vi "SA_OUT.vi"(8 "error in (no error)":errorcluster, 10 "拍攝A讀取條碼":string, 11 "DBLink":string) -> (0 "error out":errorcluster, 2 "Workspace: screw_B":cluster{"條碼A":string, "條碼B":string}[](array[cluster]), 3 "Workspace: screw_A":cluster{"條碼A":string, "條碼B":string}[](array[cluster]))   [LabVIEW 2019]
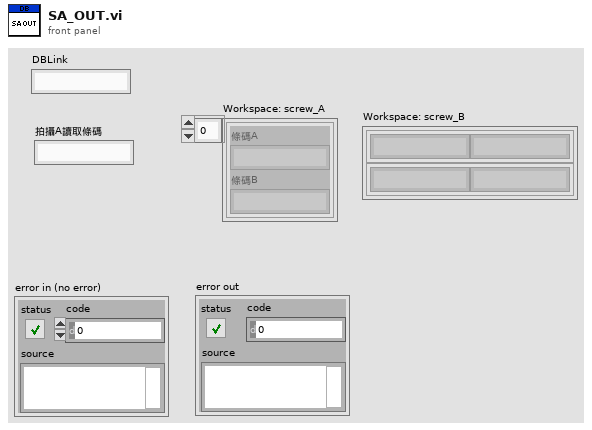
[diagram p1: front panel]
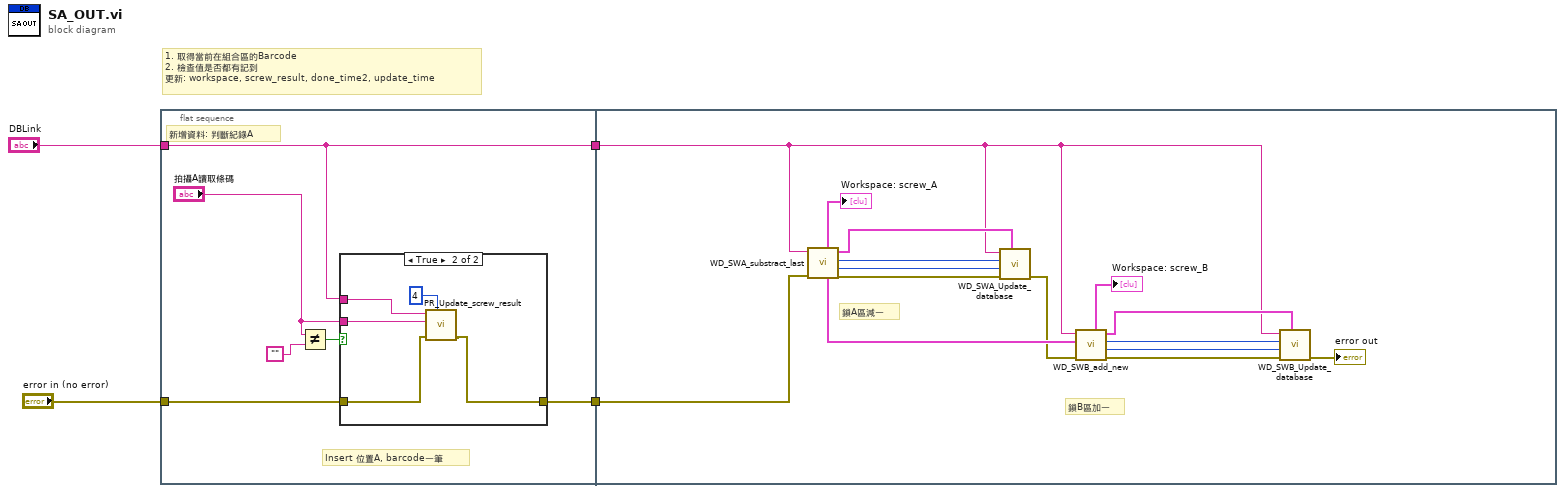
[diagram p0: block diagram]
diagram:
  # "1. 取得當前在組合區的Barcode\n2. 檢查值是否都有記到\n更新: workspace, screw_result, done_time2, update_time"
  n1 = flat-sequence {
    tunnel: "DBLink" -> [w6]
    tunnel: "error in (no error)" -> [w8]
    tunnel: [w6] -> w2
    tunnel: [w5] -> w1
    tunnel: w2 -> [w17]
    tunnel: w1 -> [w21]
    frame #0 {
      # "Insert 位置A, barcode一筆"
      # "新增資料: 判斷紀錄A"
      n2 = Not Equal?(x="拍攝A讀取條碼", y="") -> (x != y?=w9:bool)
      n3 = case shown="True" w9 {
        tunnel: w6 -> [_ w16]
        tunnel: "拍攝A讀取條碼" -> [_ w15]
        tunnel: w8 -> [w11 w14]
        tunnel: [w11 w13] -> w5
        frame False {
        }
        frame True {
          n4 = call "PR_Update_screw_result .vi"("workspace_id"=i16 4 ("workspace"), "error in (no error)"=w14, "barcode"=w15, "DBlink"=w16) -> ("error out"=w13:errorcluster)  [unwired: 7 in]
        }
      }
    }
    frame #1 {
      # "鎖A區減一"
      # "鎖B區加一"
      n5 = call "WD_SWA_substract_last.vi"("error in (no error)"=w21, "DBLink"=w17) -> ("error out"=w29:errorcluster, "站點總數"=w30:i32, "當前料數"=w31:i32, "計算用 array"=w28:cluster{"條碼A":string, "條碼B":string}[], "取出element"=w27:cluster{"條碼A":string, "條碼B":string}, "顯示用array"=→"Workspace: screw_A":cluster{"條碼A":string, "條碼B":string}[])  [unwired: 4 in]
      n6 = call "WD_SWA_Update_database.vi"("計算用array"=w28, "error in (no error)"=w29, "站點總數"=w30, "當前料數"=w31, "DBLink"=w17) -> ("error out"=w18:errorcluster)  [unwired: 6 in]
      n7 = call "WD_SWB_add_new.vi"("error in (no error)"=w18, "New data"=w27, "DBLink"=w17) -> ("error out"=w26:errorcluster, "站點總數"=w25:i32, "當前料數"=w24:i32, "計算用 array"=w23:cluster{"條碼A":string, "條碼B":string}[], "顯示用array"=→"Workspace: screw_B":cluster{"條碼A":string, "條碼B":string}[])  [unwired: 4 in]
      n8 = call "WD_SWB_Update_database.vi"("計算用array"=w23, "error in (no error)"=w26, "站點總數"=w25, "當前料數"=w24, "DBLink"=w17) -> ("error out"=→"error out":errorcluster)  [unwired: 6 in]
    }
  }
